vi "get limits.vi"(8 "error in (no error)":errorcluster, 9 "Power Supply In Use":T1, 10 "External Supply?":bool=TRUE, 11 "Channel #":T2) -> (0 "error out":errorcluster, 3 "output cluster":T3)   [LabVIEW 2018, in "NI PXI-4110 Programmable Power Supply Custom Device.lvlib"]
uses:
  NI PXI-4110 Programmable Power Supply Custom Device.lvlib
  4110_Channel #.ctl
  Power_Supply_In_Use.ctl
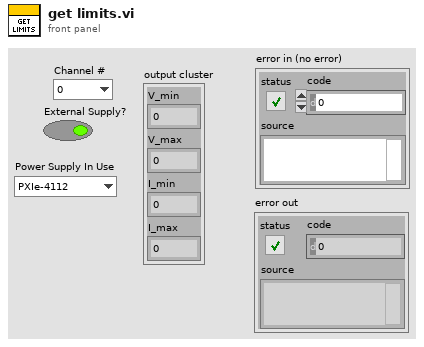
[diagram p1: front panel]
types:
  T1 = typedef "NI PXI-4110 Programmable Power Supply Custom Device.lvlib/Power_Supply_In_Use.ctl" = enum16{"PXIe-4112", "PXI-4110"}
  T2 = typedef "NI PXI-4110 Programmable Power Supply Custom Device.lvlib/4110_Channel #.ctl" = enum16{"0", "1", "2"}
  T3 = cluster{"V_min":dbl, "V_max":dbl, "I_min":dbl, "I_max":dbl}
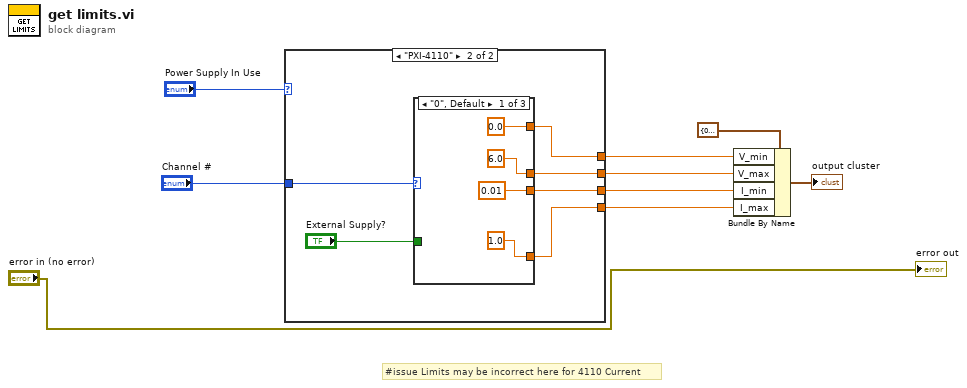
[diagram p0: block diagram]
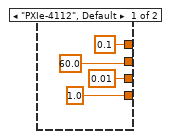
[diagram p2: hidden frame]
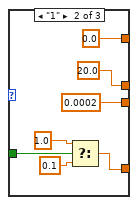
[diagram p3: hidden frame]
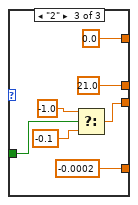
[diagram p4: hidden frame]
diagram:
  # "#issue Limits may be incorrect here for 4110 Current"
  n1 = case shown="\"PXI-4110\"" "Power Supply In Use" {
    tunnel: "Channel #" -> [_ w19]
    tunnel: [1.0 ("V_min") w18] -> w7
    tunnel: [0.01 ("V_min") w17] -> w6
    tunnel: [60.0 ("V_min") w16] -> w5
    tunnel: [0.1 ("V_min") w15] -> w4
    frame "PXIe-4112", Default {
    }
    frame "PXI-4110" {
      n2 = case shown="\"0\", Default" w19 {
        tunnel: [0.0 ("V_min") 0.0 ("V_min") 0.0 ("V_min")] -> w15
        tunnel: [6.0 ("V_min") 20.0 ("V_min") 21.0 ("V_min")] -> w16
        tunnel: [0.01 ("V_min") 0.0002 ("V_min") w32] -> w17
        tunnel: [1.0 ("V_min") w24 -0.0002 ("V_min")] -> w18
        tunnel: "External Supply?" -> [_ w27 w31]
        frame "0", Default {
        }
        frame "1" {
          n3 = Select(t=1.0, s=w27, f=0.1 ("V_min")) -> (s? t:f=w24:dbl)
        }
        frame "2" {
          n4 = Select(t=-1.0, s=w31, f=-0.1 ("V_min")) -> (s? t:f=w32:dbl)
        }
      }
    }
  }
  n5 = Bundle By Name(cluster=T3 {"V_min"=0.0, "V_max"=0.0, "I_min"=0.0, "I_max"=0.0} ("output cluster"), "V_min"=w4, "V_max"=w5, "I_min"=w6, "I_max"=w7) -> (→"output cluster":T3)
  "error out" <- "error in (no error)"
